vi "Motherson Gap algorithm int.vi"(0 "Image Out":T2(plugin-control), 1 "Calibrated Image":T2, 2 "ROI 1":T3 {"Contours"."Type" items=["No Selection", "Point", "Line", "Rectangle", "Oval", "Polygon", "Free", "Annulus", "Unused2", "Unused3", "Broken Line", "Free Hand Line", "Rotated Rectangle"]}, 3 "ROI 2":T3 {"Contours"."Type" items=["No Selection", "Point", "Line", "Rectangle", "Oval", "Polygon", "Free", "Annulus", "Unused2", "Unused3", "Broken Line", "Free Hand Line", "Rotated Rectangle"]}, 5 "error in (no error)":errorcluster) -> (14 "Gap":sgl, 16 "output cluster":T1, 19 "error out":errorcluster)   [LabVIEW 2019, in "Algorithm.lvclass"]
uses:
  FrameworkOverrides/Algorithm.lvclass
  <vilib>/vision/NI_Vision_Development_Module.lvlib
  <vilib>/vision/Measure.llb/Edge Polarity.ctl
  <vilib>/vision/Measure.llb/Edge Options.ctl
  <vilib>/vision/Image Controls.llb/IMAQ Image.ctl
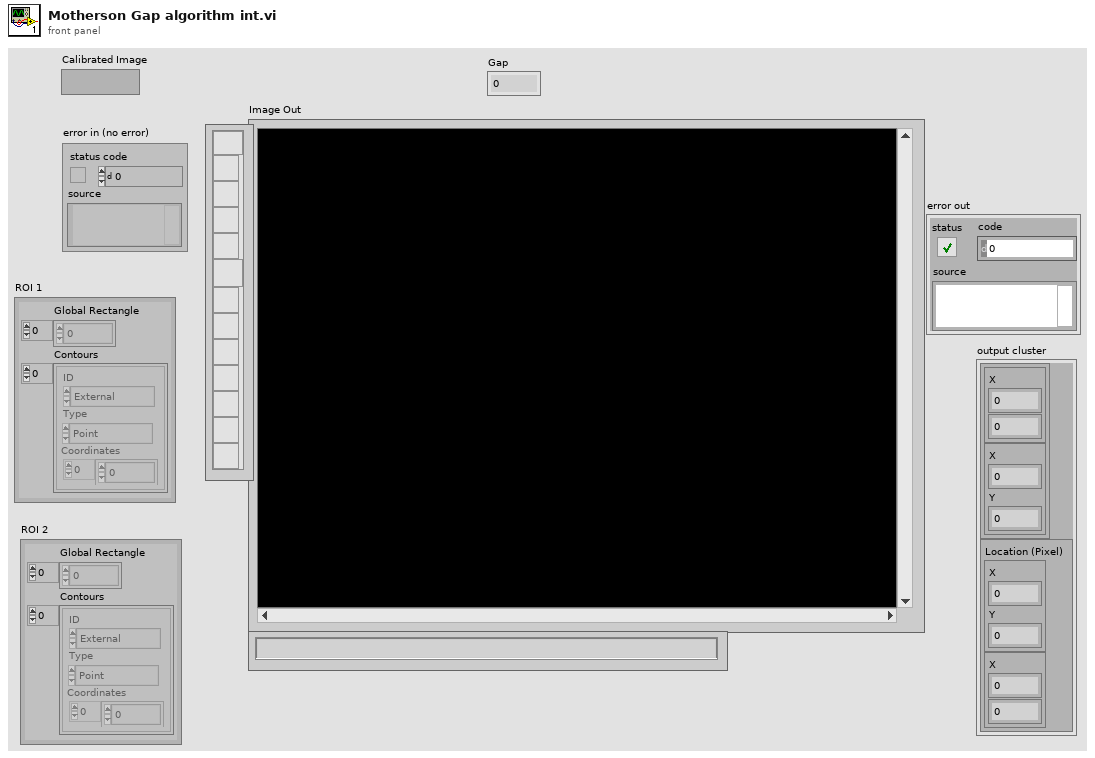
[diagram p1: front panel]
types:
  T1 = cluster{cluster{cluster{"X":sgl, sgl}, cluster{"X":sgl, "Y":sgl}}, cluster{"Location (Pixel)":cluster{"X":sgl, "Y":sgl}, cluster{"X":sgl, sgl}}}
  T2 = typedef "IMAQ Image.ctl" = refnum<image>
  T3 = cluster{"Global Rectangle":i32[], "Contours":cluster{"ID":enum32{"External", "Internal"}, "Type":u32, "Coordinates":i32[]}[]}
  T4 = enum16{"Get First Edge", "Get First + Last Edge", "Get All Edges", "Get Best Edge"}
  T5 = typedef "Edge Options.ctl" = cluster{"Edge Polarity":T6, "Kernel Size":u32, "Width":u32, "Minimum Edge Strength":sgl, "Interpolation Type":enum32{"Zero Order", "Bilinear", "Quadratic", "Cubic", "Bilinear Fixed"}, "Data Processing Method":enum32{"Average", "Median"}}
  T6 = typedef "Edge Polarity.ctl" = u32
  T7 = typedef "Edge New.ctl" = cluster{"Location (Pixel)":cluster{"X":sgl, "Y":sgl}, "Location (Real-World)":cluster{"X":sgl, "Y":sgl}, "Distance (Pixel)":dbl, "Distance (Real-World)":dbl, "Strength":dbl, "Noise":dbl, "Rising?":bool}
  T8 = cluster{cluster{"X":sgl, sgl}, cluster{"X":sgl, "Y":sgl}}
  T9 = cluster{"Location (Pixel)":cluster{"X":sgl, "Y":sgl}, cluster{"X":sgl, sgl}}
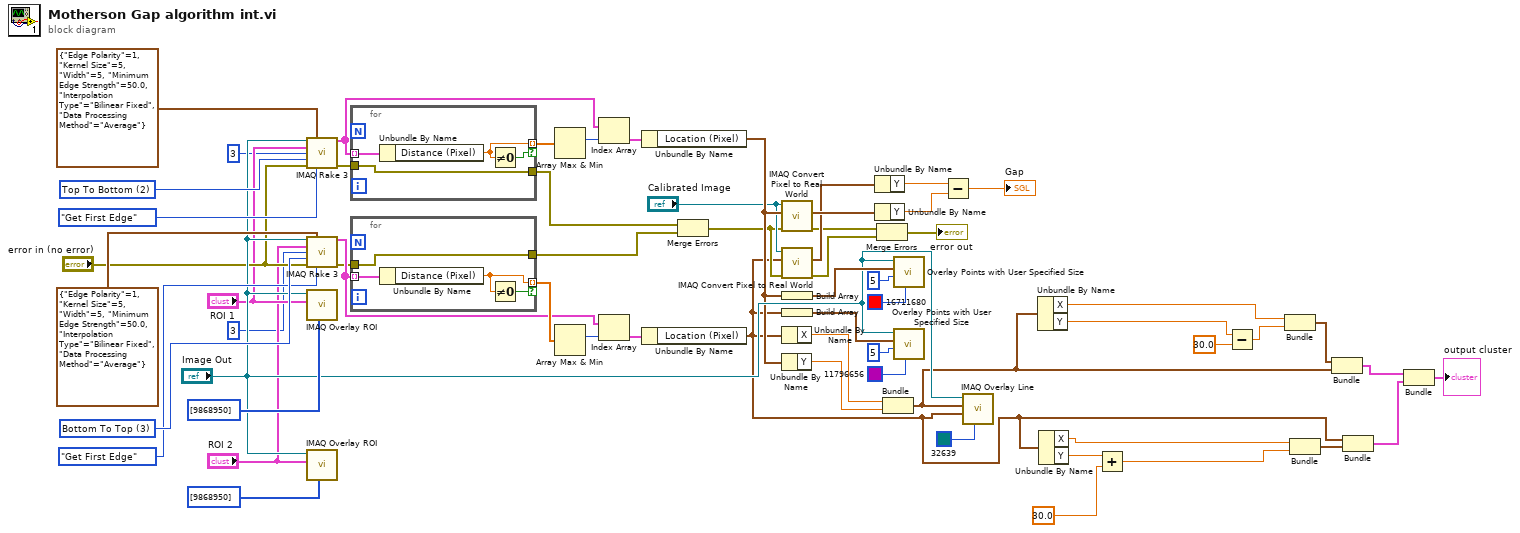
[diagram p0: block diagram]
diagram:
  w50 = u16 3 items=["Left To Right", "Right To Left", "Top To Bottom", "Bottom To Top"] ("Scan Direction")
  w60 = u16 2 items=["Left To Right", "Right To Left", "Top To Bottom", "Bottom To Top"] ("Scan Direction")
  n1 = call "IMAQ Rake 3"("Image"="Image Out", "Edge Options"=T5 {"Edge Polarity"=1, "Kernel Size"=5, "Width"=5, "Minimum Edge Strength"=50.0, "Interpolation Type"=enum."Bilinear Fixed", "Data Processing Method"=enum."Average"}, "ROI Descriptor"="ROI 1", "Step Size"=u32 3, "Scan Direction"=w60, "error in (no error)"="error in (no error)", "Process"=T4."Get First Edge") -> ("First Edges"=w56:T7[], "error out"=w52:errorcluster)  [unwired: 5 in, 2 out]
  n2 = call "IMAQ Rake 3"("Image"="Image Out", "Edge Options"=T5 {"Edge Polarity"=1, "Kernel Size"=5, "Width"=5, "Minimum Edge Strength"=50.0, "Interpolation Type"=enum."Bilinear Fixed", "Data Processing Method"=enum."Average"}, "ROI Descriptor"="ROI 2", "Step Size"=u32 3, "Scan Direction"=w50, "error in (no error)"="error in (no error)", "Process"=T4."Get First Edge") -> ("First Edges"=w43:T7[], "error out"=w42:errorcluster)  [unwired: 5 in, 2 out]
  n3 = call "IMAQ Overlay ROI"("Colors (Green)"=u32[] [9868950], "ROI Descriptor"="ROI 1", "Image"="Image Out") -> ()  [unwired: 7 in, 2 out]
  n4 = call "IMAQ Overlay ROI"("Colors (Green)"=u32[] [9868950], "ROI Descriptor"="ROI 2", "Image"="Image Out") -> ()  [unwired: 7 in, 2 out]
  n5 = for {
    tunnel: w56 -> [w65] mode=indexing
    tunnel: [w64] -> w57 mode=indexing if=w63
    tunnel: w52 -> [w62]
    tunnel: [w62] -> w41
    n6 = Unbundle By Name(w65) -> ("Distance (Pixel)"=w64:dbl)
    n7 = Not Equal To 0?(x=w64) -> (x != 0?=w63:bool)
  }
  n8 = for {
    tunnel: w43 -> [w69] mode=indexing
    tunnel: [w68] -> w47 mode=indexing if=w67
    tunnel: w42 -> [w66]
    tunnel: [w66] -> w40
    n9 = Unbundle By Name(w69) -> ("Distance (Pixel)"=w68:dbl)
    n10 = Not Equal To 0?(x=w68) -> (x != 0?=w67:bool)
  }
  n11 = Array Max & Min(array=w57) -> (max index (indices)=w51:i32)  [unwired: 3 out]
  n12 = Array Max & Min(array=w47) -> (max index (indices)=w34:i32)  [unwired: 3 out]
  n13 = Index Array(array=w56, index=w51) -> (element=w55:T7)
  n14 = Index Array(array=w43, index=w34) -> (element=w44:T7)
  n15 = Unbundle By Name(w55) -> ("Location (Pixel)"=w29:cluster{"X":sgl, "Y":sgl})
  n16 = Unbundle By Name(w44) -> ("Location (Pixel)"=w3:cluster{"X":sgl, "Y":sgl})
  n17 = Merge Errors(w41, w40) -> (w25:errorcluster)
  n18 = call "IMAQ Convert Pixel to Real World"("error in (no error)"=w25, "Pixel Coordinates"=w29, "Calibrated Image"="Calibrated Image") -> ("error out"=w24:errorcluster, "Real World Coordinates"=w27:cluster{"X":sgl, "Y":sgl})  [unwired: 3 in, 4 out]
  n19 = call "IMAQ Convert Pixel to Real World"("error in (no error)"=w25, "Pixel Coordinates"=w3, "Calibrated Image"="Calibrated Image") -> ("error out"=w23:errorcluster, "Real World Coordinates"=w26:cluster{"X":sgl, "Y":sgl})  [unwired: 3 in, 4 out]
  n20 = Build Array(w29) -> (w54:cluster{"X":sgl, "Y":sgl}[])
  n21 = Build Array(w3) -> (w45:cluster{"X":sgl, "Y":sgl}[])
  n22 = Unbundle By Name(w3) -> ("X"=w16:sgl)
  n23 = Unbundle By Name(w29) -> ("Y"=w38:sgl)
  n24 = Unbundle By Name(w26) -> ("Y"=w20:sgl)
  n25 = Unbundle By Name(w27) -> ("Y"=w19:sgl)
  n26 = Merge Errors(w24, w23) -> (→"error out":errorcluster)
  n27 = Bundle("X"=w16, "Y"=w38) -> (w14:cluster{"X":sgl, "Y":sgl})  [unwired: 1 in]
  n28 = call "Overlay Points with User Specified Size.vi"("Color"=u32 16711680, "Point Diameter (5)"=u32 5, "Points"=w54, "Image In"="Image Out") -> ()  [unwired: 6 in, 2 out]
  n29 = call "Overlay Points with User Specified Size.vi"("Color"=u32 11796656, "Point Diameter (5)"=u32 5, "Points"=w45, "Image In"="Image Out") -> ()  [unwired: 6 in, 2 out]
  n30 = Subtract(x=w20, y=w19) -> (x-y=→"Gap":sgl)
  n31 = call "IMAQ Overlay Line"("Color"=u32 32639, "End Point"=w3, "Start Point"=w14, "Image"="Image Out") -> ()  [unwired: 6 in, 2 out]
  n32 = Unbundle By Name(w14) -> ("X"=w11:sgl, "Y"=w13:sgl)
  n33 = Unbundle By Name(w3) -> ("X"=w6:sgl, "Y"=w9:sgl)
  n34 = Add(x=w9, y=sgl 30.0) -> (x+y=w7:sgl)
  n35 = Subtract(x=w13, y=sgl 30.0) -> (x-y=w12:sgl)
  n36 = Bundle("X"=w11, w12) -> (w10:cluster{"X":sgl, sgl})  [unwired: 1 in]
  n37 = Bundle("X"=w6, w7) -> (w4:cluster{"X":sgl, sgl})  [unwired: 1 in]
  n38 = Bundle(w10, w14) -> (w5:T8)  [unwired: 1 in]
  n39 = Bundle("Location (Pixel)"=w3, w4) -> (w2:T9)  [unwired: 1 in]
  n40 = Bundle(w5, w2) -> (→"output cluster":T1)  [unwired: 1 in]
